vi "SDCP FTOR Test.vi"() -> ()   [LabVIEW 2020]
uses:
  Typedefs/SDCP - Serial Port Control - Commands.ctl
panel:
  in  "interval (ms)":u32=10
  out "Current iteration":i32
  out "Intervals (ms)":u32[](array[numeric])
  in  "Number of tries":i32
  out "Received frames":u8[][](array[numeric])
  in  "FIDs":u8[](array[numeric])
  in  "VISA resource name":refnum<visa-resource-name>="COM5"
  in  "Baud rate":u32=115200
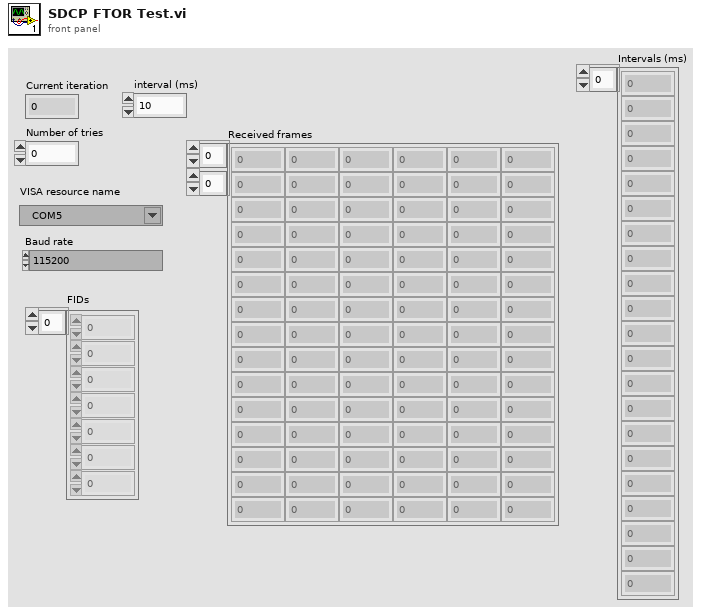
[diagram p1: front panel]
types:
  T1 = typedef "SDCP - Serial Port Control - Commands.ctl" = enum16{"Open", "Read", "Write", "Get instance", "Close"}
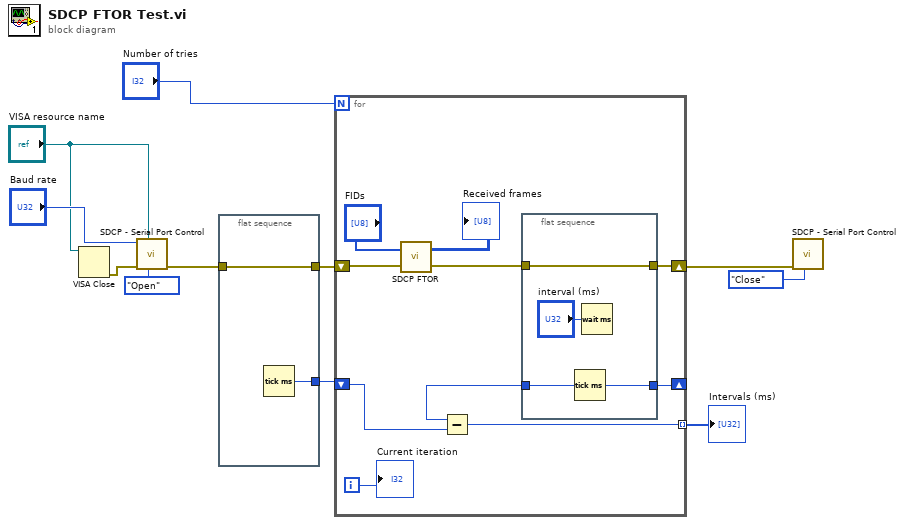
[diagram p0: block diagram]
diagram:
  n1 = VISA Close(VISA resource name="VISA resource name") -> (error out=w7:errorcluster)  [unwired: 1 in]
  n2 = call "SDCP - Serial Port Control.vi"("Command"=SDCP_-_Serial_Port_Control_-_Commands."Open", "VISA resource name"="VISA resource name", "error in (no error)"=w7, "Baud rate"="Baud rate") -> ("error out"=w2:errorcluster)  [unwired: 4 in, 3 out]
  n3 = flat-sequence {
    tunnel: [w13] -> w4
    tunnel: w2 -> [w12]
    tunnel: [w12] -> w1
    frame #0 {
      n4 = Tick Count (ms)() -> (millisecond timer value=w13:u32)
    }
  }
  n5 = for {
    N: "Number of tries" -> [_]
    shift-right: [w19] -> w9
    shift-left: w1 -> [w23]
    shift-right: [w17] -> _
    shift-left: w4 -> [w18]
    tunnel: [w15] -> w3 mode=indexing
    i -> [w14]
    n6 = call "SDCP FTOR.vi"("error in (no error)"=w23, "FID"="FIDs") -> ("error out"=w20:errorcluster, "Received frames"=→"Received frames":u8[][])
    n7 = Subtract(x=w16, y=w18) -> (x-y=w15:u32)
    n8 = flat-sequence {
      tunnel: w20 -> [w26]
      tunnel: [w26] -> w19
      tunnel: [w24] -> w17
      tunnel: [w24] -> w16
      frame #0 {
        n9 = Tick Count (ms)() -> (millisecond timer value=w24:u32)
        n10 = Wait (ms)(milliseconds to wait="interval (ms)") -> ()  [unwired: 1 out]
      }
    }
    "Current iteration" <- w14
  }
  "Intervals (ms)" <- w3
  n11 = call "SDCP - Serial Port Control.vi"("Command"=SDCP_-_Serial_Port_Control_-_Commands."Close", "error in (no error)"=w9) -> ()  [unwired: 6 in, 4 out]
